vi "BoundedFunction.vi"(1 "Input":dbl, 2 "LowerBound":dbl, 3 "UpperBound":dbl) -> (0 "Output":dbl)   [LabVIEW 2017]
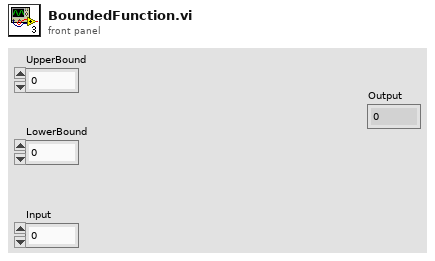
[diagram p1: front panel]
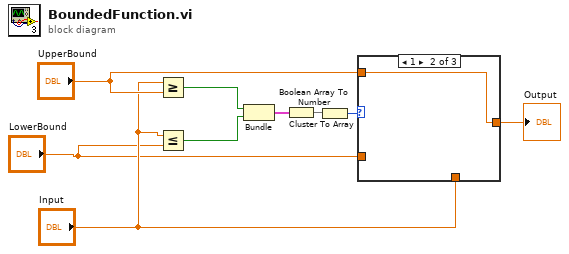
[diagram p0: block diagram]
diagram:
  n1 = Greater Or Equal?(x="Input", y="UpperBound") -> (x >= y?=w9:bool)
  n2 = Less Or Equal?(x="Input", y="LowerBound") -> (x <= y?=w8:bool)
  n3 = Bundle(w9, w8) -> (w7:cluster{bool, bool})  [unwired: 1 in]
  n4 = Cluster To Array(cluster=w7) -> (array=w6:bool[])
  n5 = Boolean Array To Number(Boolean array=w6) -> (number=w5:u32)
  n6 = case shown="1" w5 {
    tunnel: [w10 w11 w12] -> w4
    tunnel: "Input" -> [w10 _ _]
    tunnel: "UpperBound" -> [_ w11 _]
    tunnel: "LowerBound" -> [_ _ w12]
    frame 0, Default {
    }
    frame 1 {
    }
    frame 2 {
    }
  }
  "Output" <- w4
